vi "DashboardClientUI.vi"() -> ()   [LabVIEW 2017, in "Client.lvlib"]
uses:
  Client.lvlib
panel:
  in  "Stop":bool
  out "Connection Quality":dbl(knob) scale=0.0..10.0
  out "Connected?":bool
  out "Last Update":timestamp
  in  "OK Button":bool
  in  "Vertical Refresh Button":bool
  in  "AE Level":enum16{"AE / ELP", "AE Intern"}(ring)
  in  "AE Groups":i32(listbox)
  in  "SRs Tab":T1(tab)
  in  "Unassigned SRs":string(tree)
  in  "Save Unassigned":bool
  in  "Save Unassigned 2":bool
  in  "Assigned SRs":string(tree)
  out "error out":errorcluster
  in  "DecorationControl":i32(listbox)
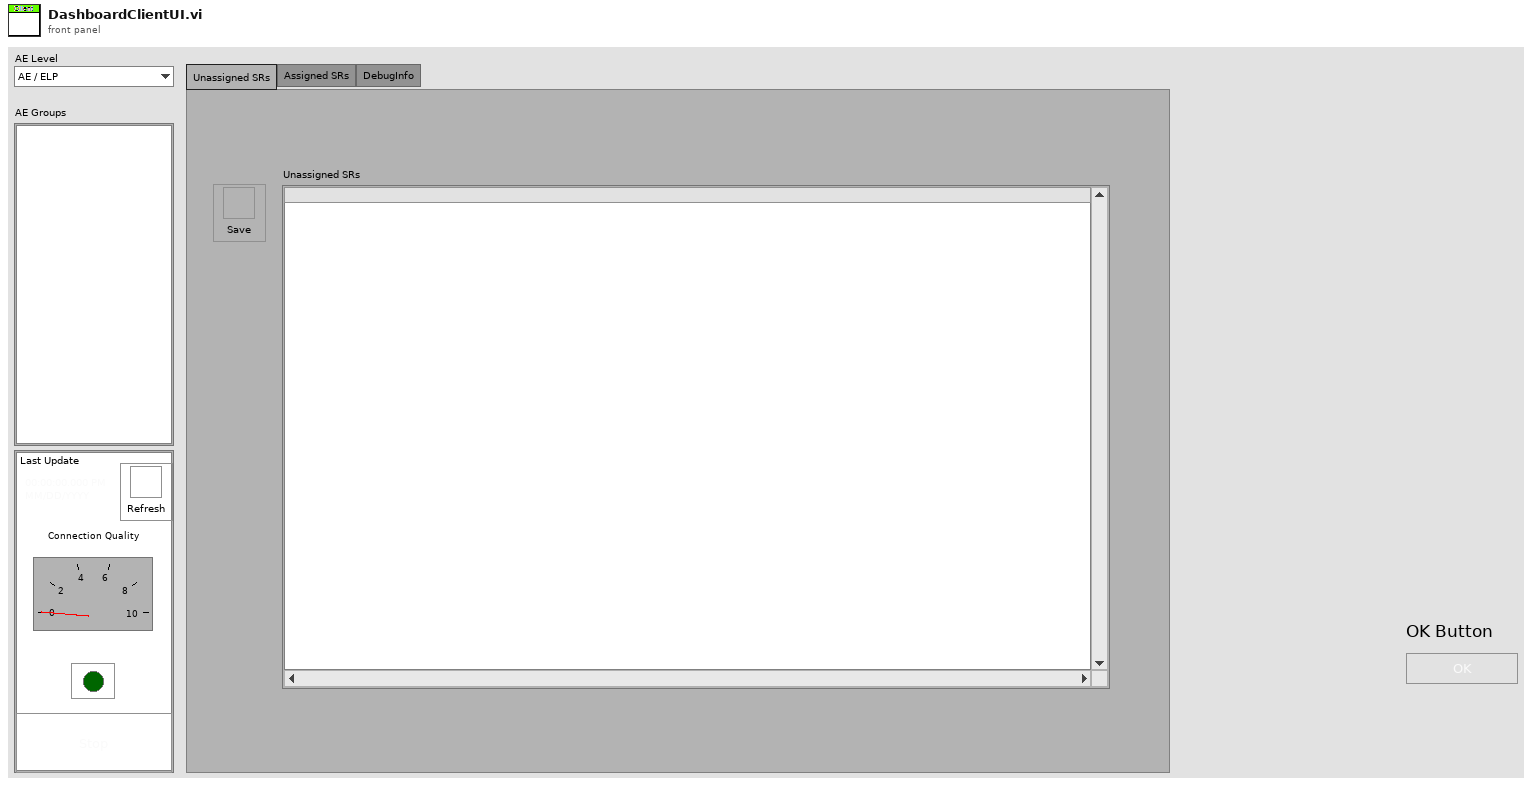
[diagram p1: front panel]
types:
  T1 = enum32{"Unassigned SRs", "Assigned SRs", "DebugInfo"}
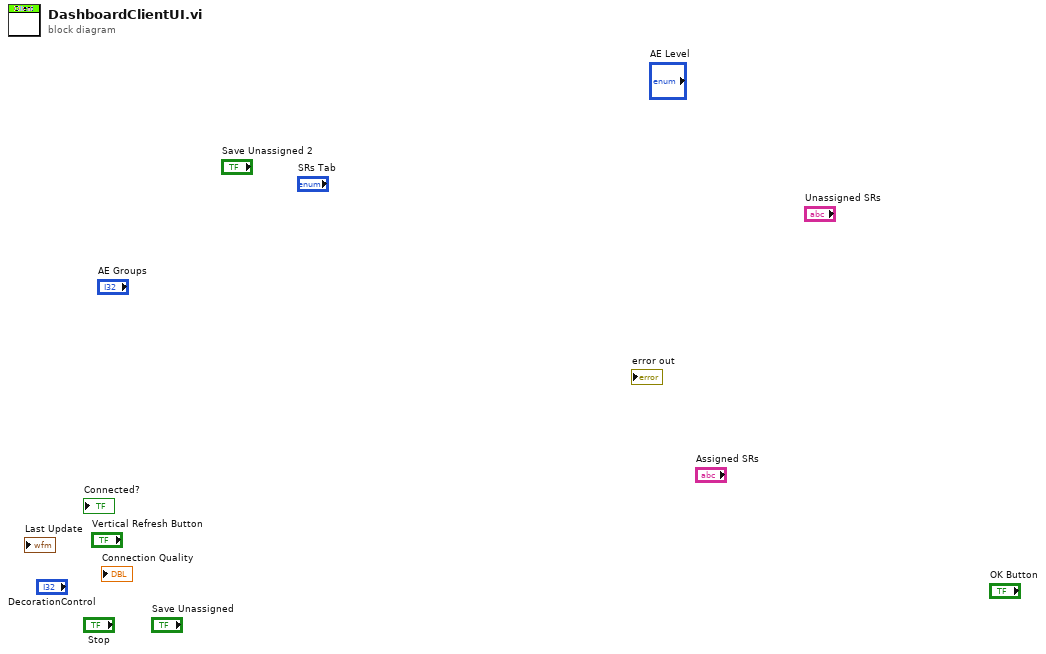
[diagram p0: block diagram]
diagram:
